vi "Window-Functional data editor.vi"(9 "Experiment Path":path=path "C:/Users/Teo/Desktop/UCL Datasets/160915_13_48_57 FunctAcq-6 patches", 11 "Standalone viewer?":bool=TRUE) -> ()   [LabVIEW 2020]
uses:
  User Interface/Visualisation/Timelapse Viewer/Typedefs/Custom slider-vertical.ctl
  User Interface/Visualisation/Timelapse Viewer/Typedefs/Colour.ctl
  User Interface/Visualisation/Timelapse Viewer/Typedefs/Channel to load.ctl
  User Interface/Visualisation/Timelapse Viewer/Typedefs/Time series viewer refs.ctl
  User Interface/Visualisation/Timelapse Viewer/Typedefs/Speed Viewer States enum.ctl
  <vilib>/Utility/miscctls.llb/LVPointTypeDef.ctl
  Typedefs/Save-Load enum.ctl
  <vilib>/vision/Image Controls.llb/IMAQ Image.ctl
  Typedefs/HW config states enum.ctl
  User Interface/Visualisation/Functional Imaging Viewer/Typedefs/Get-Set-Clear Control.ctl
  User Interface/Visualisation/Timelapse Viewer/Typedefs/Select Play-Stop button to show.ctl
  <vilib>/Utility/error.llb/DialogType.ctl
  User Interface/Visualisation/Timelapse Viewer/Cam video sync/Typedefs/Cam videos cluster.ctl
  User Interface/Visualisation/Timelapse Viewer/Globals/gl_Time series viewer globals.vi
  Global Variables/General Globals.vi
panel:
  in  "Channel to load":T1
  in  "Colour":T2
  in  "Number of rows to generate":i32=3 format="%.0f rows"
  in  "Source number of frames":T3(ring)=enum."As many as the number of cycles"
  out "Slider at frame #":i32 format="Cycle %.0f"
  in  "Scrollbar":i32(c297)
  in  "Back":bool
  in  "Play":bool
  in  "Stop":bool
  in  "Tab Control":enum32{"Camera videos", "Speed data"}(tab)
  out "Cams":T5 {"Vid4 Rel time (ms)" format="%.0f ms"; "Vid3 Rel time (ms)" format="%.0f ms"; "Vid2 Rel time (ms)" format="%.0f ms"; "Vid1 Rel time (ms)" format="%.0f ms"}
  out "Actual number \nof speed points":i32 format="Actual of speed points: %.0f"
  out "Speed Data":string[][](array[string])
  out "Expected speed values":dbl format="Expected speed points: %#_g"
  out "Original frame rate (fps)":dbl format="Original frame rate: %#.1f (fps)"
  out "Frame rate set (fps)":dbl format="Frame rate set: %#.1f (fps)"
  out "Actual frame rate (fps)":dbl format="Actual frame rate: %#.1f (fps)"
  out "AVI Mode ind":string="AVI mode:"
  out "Video length info":string="Duration: 00h 00m 00s, 0 frames"
  out "Export images":bool
  out "Export snippet":bool
  in  "Extraction Cursors":cluster{i32, i32}(slide)={1, 5594} scale=1.0..141.0
  out "Export vid":bool
  out "Stop (ind)":bool
  in  "Intensity":T6={0.0, 4095.0} scale=0.0..4095.0
  out "Speed Graph":dbl[](graph) caption="Speed Chart"
  out "Image":T4(plugin-control)
  # "Date                         Time                  Time stamp           Speed (rpm)          Angle (deg)"
  # "Timelapse Info"
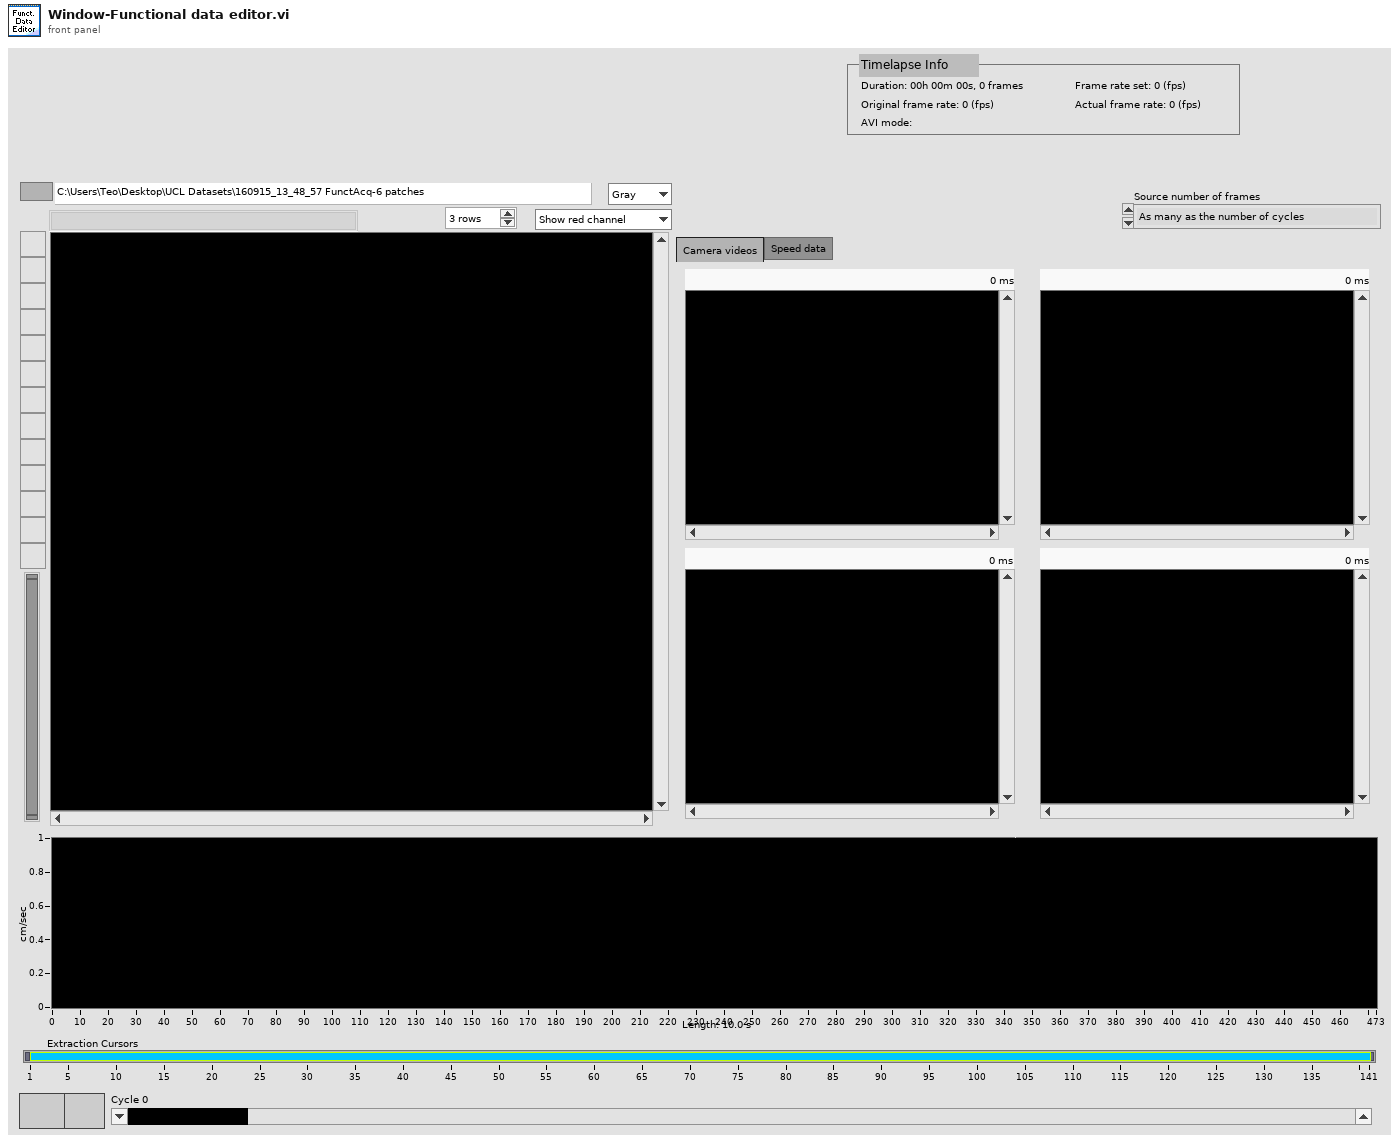
[diagram p1: front panel]
types:
  T1 = typedef "Channel to load.ctl" = enum16{"Show red channel", "Show green channel", "Show both channels"}
  T2 = typedef "Colour.ctl" = enum16{"Gray", "Red", "Green", "Mixed"}
  T3 = enum16{"As many as the frames in the video with the fewest frames", "As many as the number of cycles"}
  T4 = typedef "IMAQ Image.ctl" = refnum<image>
  T5 = cluster{"Vid 1":T4, "Vid 2":T4, "Vid 3":T4, "Vid 4":T4, "Vid1 Rel time (ms)":u32, "Vid2 Rel time (ms)":u32, "Vid3 Rel time (ms)":u32, "Vid4 Rel time (ms)":u32}
  T6 = typedef "Custom slider-vertical.ctl" = cluster{dbl, dbl}
  T7 = typedef "Time series viewer refs.ctl" = cluster{"This VI":refnum<vi>, "Image control":refnum<vi>, "AVI Mode ind":refnum<vi>, "Play":refnum<vi>, "Stop":refnum<vi>, "Back":refnum<vi>, "Scrollbar":refnum<vi>, "Video length info":refnum<vi>, "Expected speed values":refnum<vi>, "Intensity":refnum<vi>, "Path":refnum<vi>, "Selection sliders":refnum<vi>, "Speed Graph ref":refnum<vi>, "Frame rate set (fps)":refnum<vi>, "Number of rows to generate":refnum<vi>, "VL Image Array":refnum<vi>, "Image Scrollbar":refnum<vi>, "Channel to load":refnum<vi>, "Colour":refnum<vi>}
  T8 = typedef "Save-Load enum.ctl" = enum16{"Save to file", "Load from file", "Compare from file", "Save Backup"}
  T9 = enum16{"None", "Release queue", "Obtain queue", "Enqueue", "Get status", "Set status"}
  T10 = typedef "LVPointTypeDef.ctl" = cluster{"Horizontal":i16, "Vertical":i16}
  T11 = typedef "Speed Viewer States enum.ctl" = enum16{"Idle", "Initialise", "Playback", "Scroll bar event", "Speed cursor event", "Back to start", "Exit"}
  T12 = typedef "HW config states enum.ctl" = enum16{"Load from file", "Save to file", "Save backup", "Write all", "Read all", "Write XY stage settings", "Write DAQ FPGA settings", "Write Control FPGA settings", "Write Phys Channels", "Write System Config", "Write HW Config", "Save System Config", "Save HW Config", "Clear", "Compare from file"}
  T13 = typedef "Image Type" = u32
  T14 = typedef "Custom slider-horisontal.ctl" = cluster{dbl, dbl}
  T15 = typedef "Cam videos cluster.ctl" = cluster{"Vid 1":T4, "Vid 2":T4, "Vid 3":T4, "Vid 4":T4, "Vid1 Rel time (ms)":u32, "Vid2 Rel time (ms)":u32, "Vid3 Rel time (ms)":u32, "Vid4 Rel time (ms)":u32}
  T16 = typedef "Get-Set-Clear Control.ctl" = enum16{"Get", "Set", "Clear"}
  T17 = typedef "Select Play-Stop button to show.ctl" = enum16{"Show Play button", "Show Stop button"}
  T18 = typedef "DialogType.ctl" = u16
  T19 = typedef "Hardware Configuration settings.ctl" = cluster{"Dev. PC":bool, "Swap XY on stage":bool, "No of AOD":u8, "MC Supported":bool, "Axial MC":bool, "Computer MAC address":string, "Externalise Triggers":bool, "Trigger HW config":T20, "DAQmx Chan":T21, "XY stage available":bool, "XY Stage":T22, "Z stage available":bool, "Z Stage config cluster":T23, "Encoder available":bool, "Encoder":T24, "VidRec available":bool, "Cam VidRec":T25, "Laser Power Control HW config":T26, "Laser 1 available":bool, "Laser 1 config cluster":T27, "Prechirper 1 available":bool, "Prechirper 1 config cluster":T28, "Control system.FPGA available?":bool, "Control Sys. HW config":T29, "DAQ FPGA HW Config":T30, "PMT Voltage Range":T34}
  T20 = typedef "Triggers HW config.ctl" = cluster{"Available Device List":i32, "Device Address":string}
  T21 = typedef "DAQmx physical channels cluster.ctl" = cluster{"Pockels AO":tag, "Hard shutter AO":tag, "PMT AOs":tag, "Galvo AOs":tag, "Power meter AI":tag}
  T22 = typedef "XY Stage config cluster.ctl" = cluster{"COM port":refnum<visa-resource-name>, "Baudrate":i32, "Type":string}
  T23 = typedef "Z Stage config cluster.ctl" = cluster{"COM port":refnum<visa-resource-name>, "Baudrate":i32, "Type":string}
  T24 = typedef "Encoder config cluster.ctl" = cluster{"IP address":string, "Port":u16, "Wheel radius (cm)":dbl, "Encoder Trigger":tag}
  T25 = typedef "Cam VidRec HW config setup cluster.ctl" = cluster{"DO flag-Video record":tag, "DO flag-Trial start":tag}
  T26 = typedef "Laser Power Control HW config.ctl" = cluster{"Laser Power Control":string, "Laser Power Modulation Control":enum16{"NI", "FPGA"}}
  T27 = typedef "Laser 1 config cluster.ctl" = cluster{"COM port":refnum<visa-resource-name>, "Baud Rate":i32, "Type":string}
  T28 = typedef "PreChirper 1 config cluster.ctl" = cluster{"Type":string, "Baud Rate":i32, "COM port":refnum<visa-resource-name>}
  T29 = typedef "Control Sys HW config cluster.ctl" = cluster{"Control system.FPGA Type":enum16{"Virtex 5", "Virtex 7"}, "Control system.Network adapter name":string, "Control system.MAC address":string, "Control system.Ethernet Port":u32, "Control system.Ethernet Port Opened":bool}
  T30 = typedef "DAQ FPGA HW config cluster.ctl" = cluster{"FGPA Ref":T31, "Target":T32, "input card type":T33}
  T31 = typedef "FPGA Ref.ctl" = refnum<k20>
  T32 = typedef "nirio_resource_hc.ctl" = tag
  T33 = typedef "FPGA input type AC-DC.ctl" = enum16{"AC Card", "DC Card"}
  T34 = typedef "PMT Voltage Range.ctl" = cluster{"PMT Voltage Lower Limit":dbl, "PMT Voltage Upper Limit":dbl}
  T35 = cluster{"Start Frame No":i32, "End Frame No":i32}
  T36 = typedef "IMAQ AVI2 Refnum.ctl" = refnum<k20>
  T37 = cluster{"# of frames to export":i32, "Initial frame's owning file":T36, "8-bit AVI file path":path, "Cursors location":cluster{"Number of first frame":i32, "Number of last frame":i32}}
  T38 = enum32{"Invalid", "Standard", "Closed", "Hidden", "Minimized", "Maximized"}
  T39 = typedef "Speed graph behaviour enum.ctl" = enum16{"Scrolling data", "Scrolling cursor"}
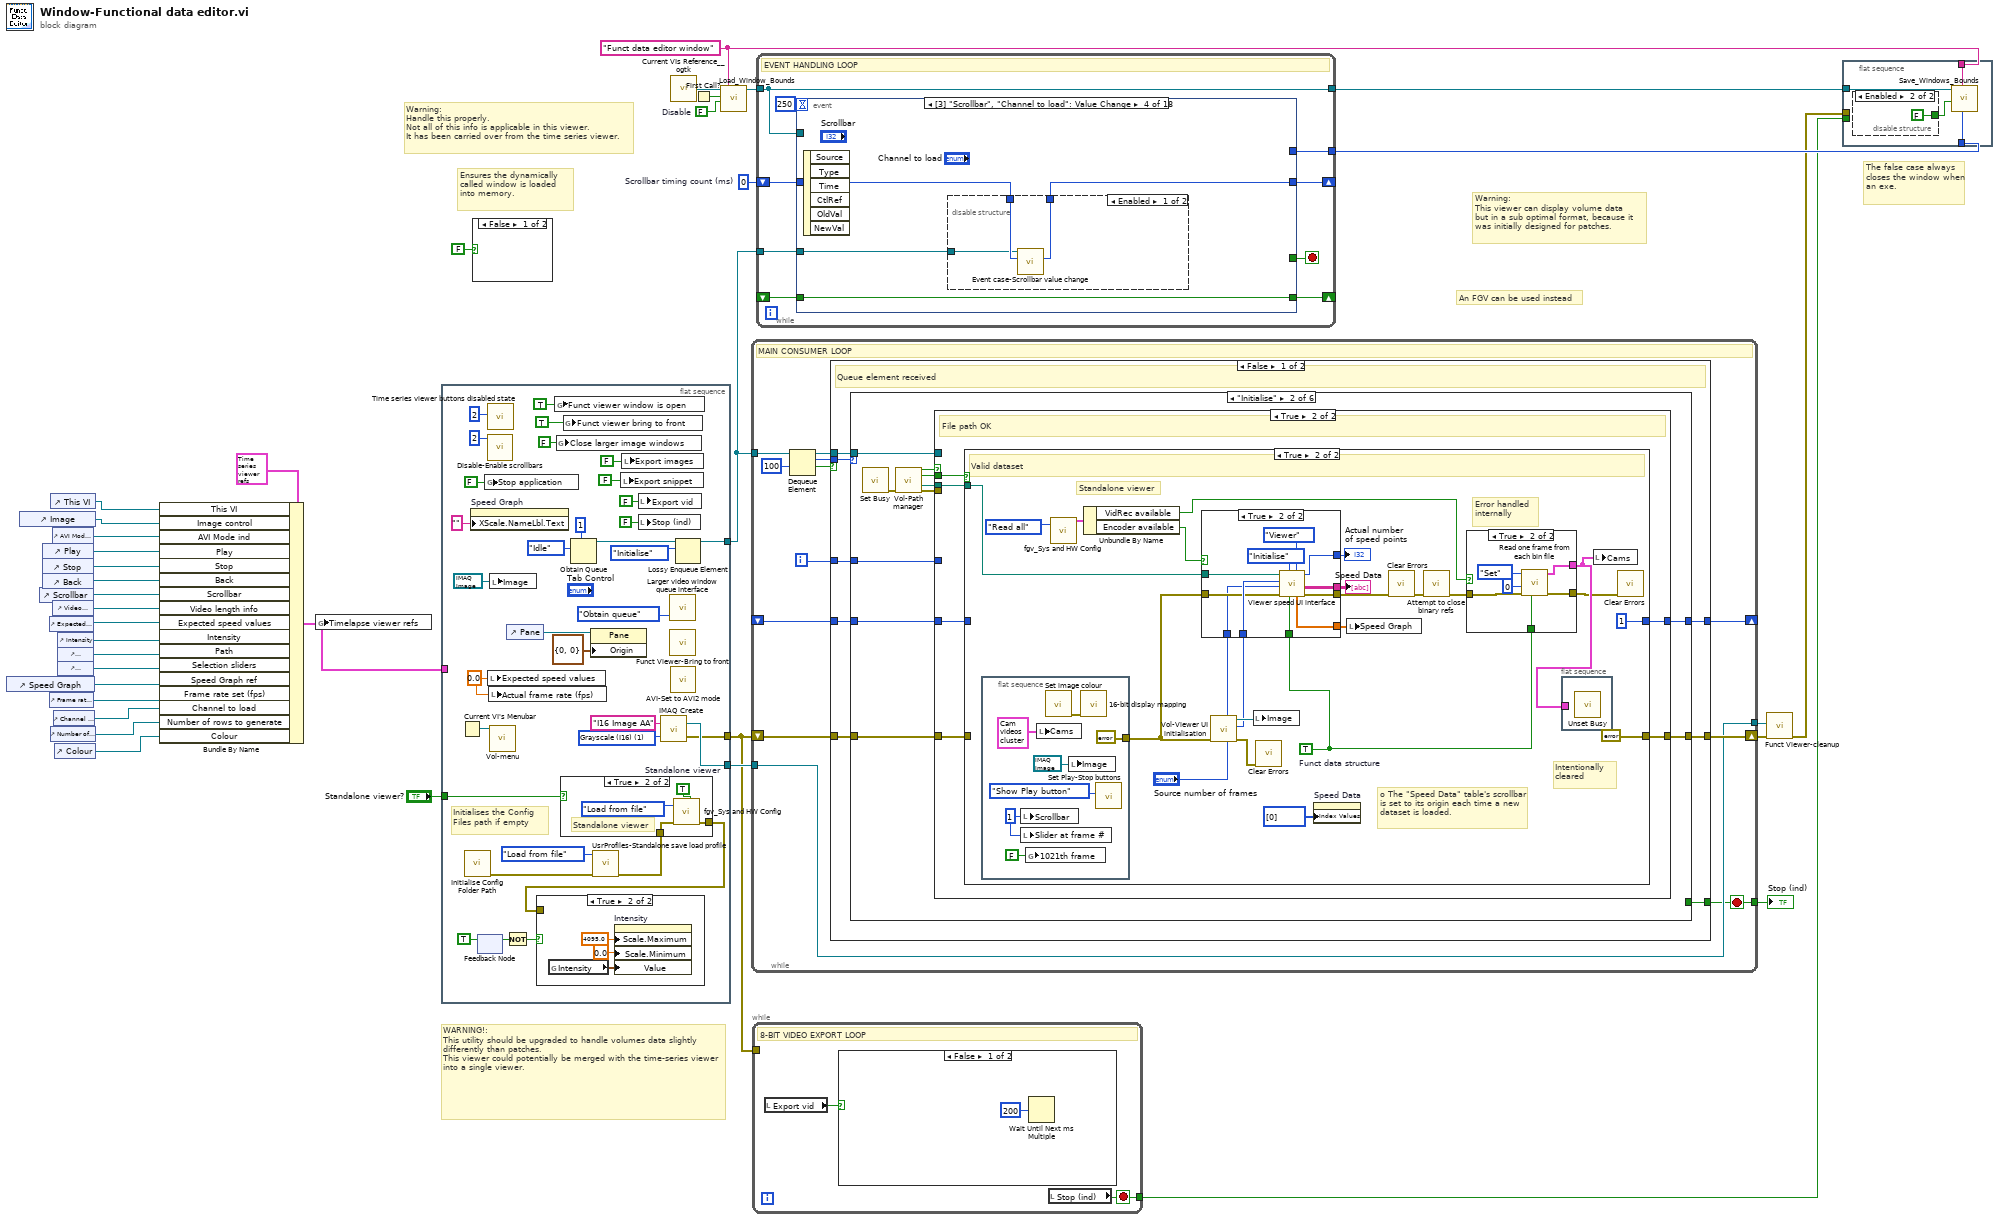
[diagram p0: block diagram]
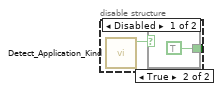
[diagram p2: hidden frame]
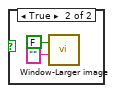
[diagram p4: hidden frame]
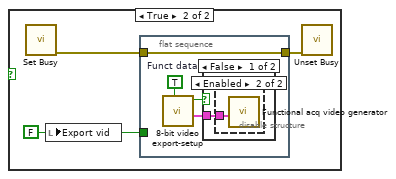
[diagram p5: hidden frame]
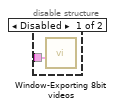
[diagram p6: hidden frame]
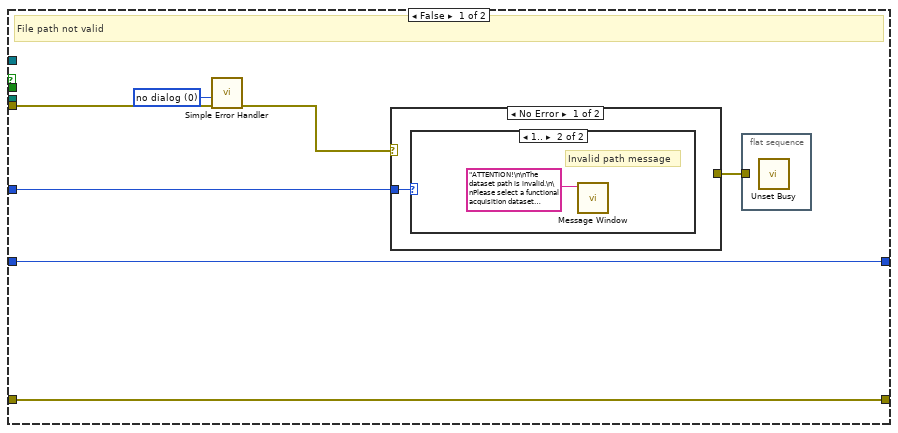
[diagram p11: hidden frame]
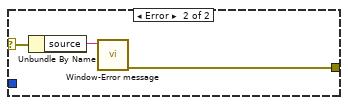
[diagram p13: hidden frame]
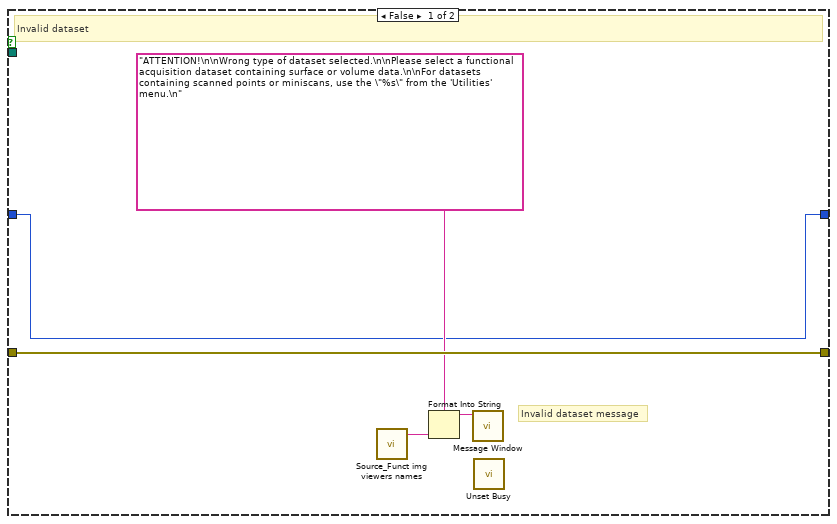
[diagram p14: hidden frame]
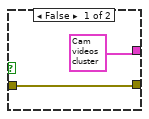
[diagram p15: hidden frame]
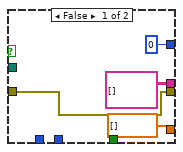
[diagram p16: hidden frame]
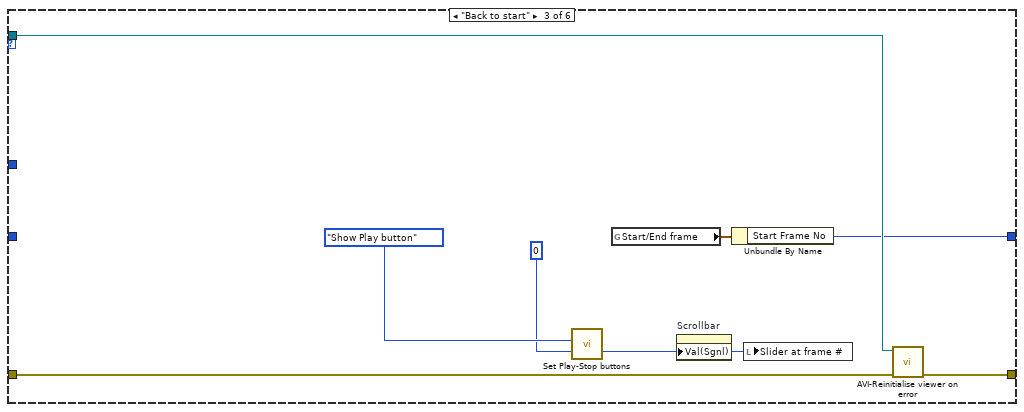
[diagram p17: hidden frame]
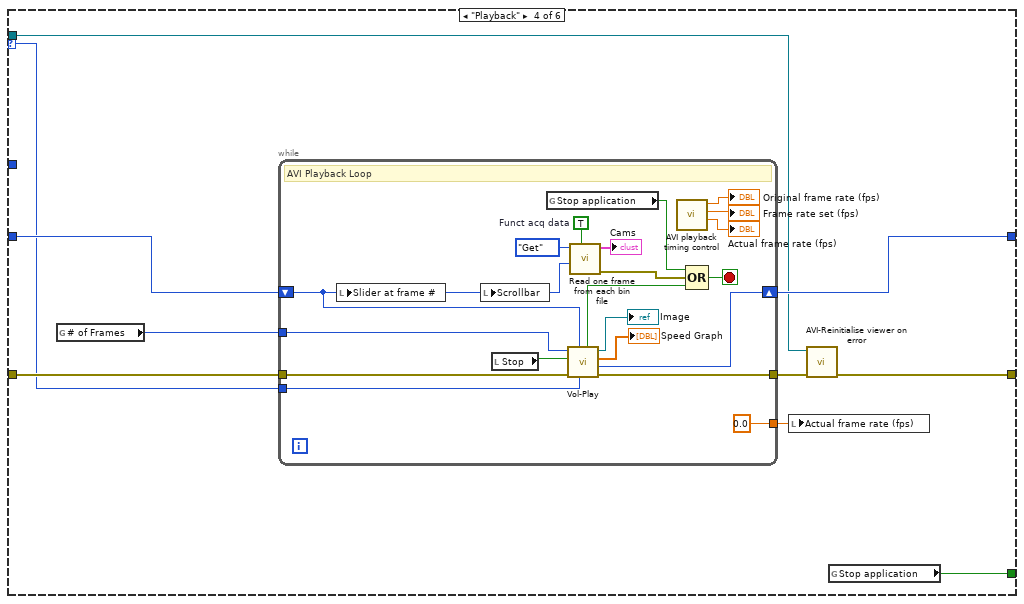
[diagram p18: hidden frame]
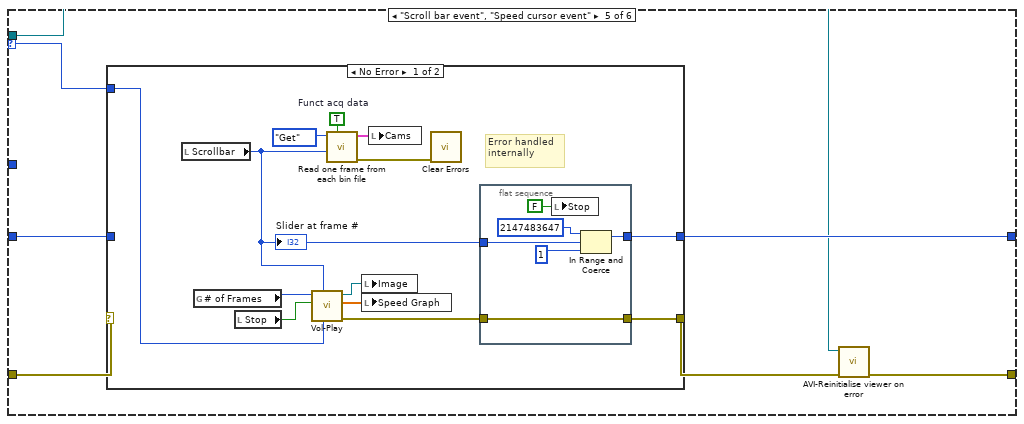
[diagram p19: hidden frame]
diagram:
  w15 = FALSE  # Disable
  w14 = "Funct data editor window" ("Window Name (i.e. Key)")
  w24 = u32 0  # Scrollbar timing count (ms)
  # "Warning:\nThis viewer can display volume data\nbut in a sub optimal format, because it\nwas initially designed for patches."
  # "Warning:\nHandle this properly.\nNot all of this info is applicable in this viewer.\nIt has been carried over from the time series viewer."
  # "WARNING!:\nThis utility should be upgraded to handle volumes data slightly differently than patches.\nThis viewer could potentially be merged with the time-series viewer into a single viewer."
  # "The false case always closes the window when an exe."
  # "Ensures the dynamically called window is loaded into memory."
  # "An FGV can be used instead"
  n1 = control-ref of="Speed Graph"() -> (w19:refnum<vi>)
  n2 = control-ref of="Image"() -> (w4:refnum<vi>)
  n3 = control-ref of="Scrollbar"() -> (w28:refnum<vi>)
  n4 = control-ref of="Play"() -> (w31:refnum<vi>)
  n5 = control-ref of="Stop"() -> (w30:refnum<vi>)
  n6 = control-ref of="Back"() -> (w29:refnum<vi>)
  n7 = control-ref of="Expected speed values"() -> (w26:refnum<vi>)
  n8 = control-ref of="Frame rate set (fps)"() -> (w8:refnum<vi>)
  n9 = control-ref of="This VI"() -> (w22:refnum<vi>)
  n10 = control-ref of="Number of rows to generate"() -> (w6:refnum<vi>)
  n11 = control-ref of="AVI Mode ind"() -> (w34:refnum<vi>)
  n12 = control-ref of="Video length info"() -> (w27:refnum<vi>)
  n13 = control-ref of="Channel to load"() -> (w2:refnum<vi>)
  n14 = control-ref of="Colour"() -> (w1:refnum<vi>)
  n15 = control-ref of="Intensity"() -> (w25:refnum<vi>)
  n16 = control-ref of="Experiment Path"() -> (w23:refnum<vi>)
  n17 = control-ref of="Extraction Cursors"() -> (w20:refnum<vi>)
  n18 = Bundle By Name(cluster=T7 {"This VI"=refnum, "Image control"=refnum, "AVI Mode ind"=refnum, "Play"=refnum, "Stop"=refnum, "Back"=refnum, "Scrollbar"=refnum, "Video length info"=refnum, "Expected speed values"=refnum, "Intensity"=refnum, "Path"=refnum, "Selection sliders"=refnum, "Speed Graph ref"=refnum, "Frame rate set (fps)"=refnum, "Number of rows to generate"=refnum, "VL Image Array"=refnum, "Image Scrollbar"=refnum, "Channel to load"=refnum, "Colour"=refnum}, "This VI"=w22, "Image control"=w4, "AVI Mode ind"=w34, "Play"=w31, "Stop"=w30, "Back"=w29, "Scrollbar"=w28, "Video length info"=w27, "Expected speed values"=w26, "Intensity"=w25, "Path"=w23, "Selection sliders"=w20, "Speed Graph ref"=w19, "Frame rate set (fps)"=w8, "Channel to load"=w2, "Number of rows to generate"=w6, "Colour"=w1) -> (w3:T7)
  n19 = global write "gl_Time series viewer globals.vi" "Timelapse viewer refs"(w3) -> ()
  n20 = flat-sequence {
    tunnel: [w69] -> w37
    tunnel: [w42] -> w18
    tunnel: [w66] -> w35
    tunnel: w3 -> [_]
    tunnel: "Standalone viewer?" -> [w41]
    frame #0 {
      w62 = 0.0 ("Expected speed points")
      w71 = T13 1 items=["Grayscale (U8)", "Grayscale (I16)", "Grayscale (SGL)", "Complex (CSG)", "RGB (U32)", "HSL (U32)", "RGB (U64)", "Grayscale (U16)"] ("Image Type")
      # "Initialises the Config Files path if empty"
      n21 = Current VI's Menubar() -> (w61:refnum<k9>)
      n22 = call "Initialise Config Folder Path.vi"() -> ("error out"=w47:errorcluster)  [unwired: 9 in, 2 out]
      n23 = property on="Speed Graph" class="WFGraph (strict)"("XScale.NameLbl.Text"="" ("X Scale.Name Label.Text")) -> ()  [unwired: 2 in, 2 out]
      n24 = feedback #1() -> (w43:bool)  [unwired: 1 in]
      n25 = feedback-in #1(TRUE) -> ()
      n26 = global write "General Globals.vi" "Stop application"(FALSE ("Stop application")) -> ()
      n27 = call "Disable-Enable scrollbars.vi"("Disabled state"=2) -> ()  [unwired: 10 in, 1 out]
      n28 = call "Time series viewer buttons disabled state.vi"("Disabled"=2) -> ()  [unwired: 10 in, 1 out]
      n29 = local write "Expected speed values"(w62) -> ()
      n30 = local write "Actual frame rate (fps)"(w62) -> ()
      n31 = local write "Image"(T4 refnum ("Image")) -> ()
      n32 = call "Vol-menu.vi"("menu"=w61) -> ()  [unwired: 9 in, 2 out]
      n33 = Not(x=w43) -> (.not. x?=w45:bool)
      n34 = control-ref of="Pane"() -> (w63:refnum<vi>)
      n35 = global write "gl_Time series viewer globals.vi" "Funct viewer window is open"(TRUE ("Bring Timelapse Editor to front")) -> ()
      n36 = global write "gl_Time series viewer globals.vi" "Close larger image windows"(FALSE ("Close larger image window")) -> ()
      n37 = global write "gl_Time series viewer globals.vi" "Funct viewer bring to front"(TRUE ("Window is open")) -> ()
      n38 = Obtain Queue(max queue size (-1, unlimited)=1, element data type=Speed_Viewer_States_enum."Idle" ("States")) -> (queue out=w67:refnum<queue>)  [unwired: 3 in, 2 out]
      n39 = property class="Pane"(reference=w63, "Origin"=T10 {"Horizontal"=0, "Vertical"=0}) -> ()  [unwired: 1 in, 2 out]
      n40 = call "UsrProfiles-Standalone save load profile.vi"("Error in"=w47, "Function"=Save-Load_enum."Load from file") -> ("error out"=w40:errorcluster)  [unwired: 9 in]
      n41 = case shown="True" w41 {
        tunnel: w40 -> [w72 w75]
        tunnel: [w72 w74] -> w39
        frame False {
          # "No need to load the system\nconfig. Already loaded."
        }
        frame True {
          w73 = TRUE  # Standalone viewer
          # "Standalone viewer"
          n42 = call "fgv_Sys and HW Config.vi"("Standalone viewer initialisation?"=w73, "Function"=HW_config_states_enum."Load from file", "error in (no error)"=w75) -> ("error out"=w74:errorcluster)  [unwired: 6 in, 2 out]
        }
      }
      n43 = case shown="True" w45 {
        tunnel: w39 -> [_ _]
        frame False {
        }
        frame True {
          n44 = global read "gl_Time series viewer globals.vi" "Intensity"() -> (w77:T14)
          n45 = property on="Intensity" class="Slide (strict)"("Scale.Maximum"=4095.0 ("Scale.Range:Maximum"), "Scale.Minimum"=0.0 ("Scale.Range:Minimum"), "Value"=w77) -> ()  [unwired: 2 in, 2 out]
        }
      }
      n46 = local write "Export snippet"(FALSE ("Export data subset")) -> ()
      n47 = local write "Export images"(FALSE ("Export data subset")) -> ()
      n48 = local write "Export vid"(FALSE ("Export")) -> ()
      n49 = local write "Stop (ind)"(FALSE ("Boolean")) -> ()
      n50 = call "IMAQ Create"("Image Name"="I16 Image AA", "Image Type"=w71) -> ("New Image"=w69:T4, "error out"=w42:errorcluster)  [unwired: 2 in, 1 out]
      n51 = call "Larger video window queue interface.vi"("Function"=T9."Obtain queue") -> ()  [unwired: 10 in, 1 out]
      n52 = call "Funct Viewer-Bring to front.vi"() -> ()  [unwired: 12 in]
      n53 = call "AVI-Set to AVI2 mode.vi"() -> ()  [unwired: 11 in, 1 out]
      n54 = Lossy Enqueue Element(queue=w67, element=Speed_Viewer_States_enum."Initialise" ("States")) -> (queue out=w66:refnum<queue>)  [unwired: 1 in, 3 out]
    }
  }
  n55 = case shown="False" FALSE {
    frame False {
    }
    frame True {
      n56 = call "Window-Larger image.vi"("Image name"="", "Open maximised"=FALSE) -> ()  [unwired: 10 in]
    }
  }
  n57 = call <userlib>:"Current VIs Reference__ogtk.vi"() -> ("Current VI's reference"=w17:refnum<vi>)  [unwired: 5 in]
  n58 = First Call?() -> (First Call?: T/F=w16:bool)
  n59 = call "Load_Window_Bounds.vi"("Window Name (i.e. Key)"=w14, "Disable"=w15, "First Call"=w16, "Window VI's Ref"=w17) -> ("reference out"=w11:refnum<vi>)  [unwired: 4 in, 3 out]
  n60 = while {
    tunnel: w37 -> [w85]
    tunnel: [w85] -> w36
    shift-right: [w91] -> _
    shift-left: _ -> [w90]
    tunnel: w35 -> [w89]
    shift-right: [w92] -> w32
    shift-left: w18 -> [w93]
    tunnel: [w84] -> w21
    i -> [w83]
    stop <- w84 stop-if-true
    # "MAIN CONSUMER LOOP"
    n61 = Dequeue Element(queue=w89, timeout in ms (-1)=100) -> (queue out=w82:refnum<queue>, element=w86:T11, timed out?=w87:bool)  [unwired: 1 in, 1 out]
    n62 = case shown="False" w87 {
      tunnel: w93 -> [w101 w262]
      tunnel: [w100 w262] -> w92
      tunnel: [w99 w263] -> w91
      tunnel: w90 -> [w98 w263]
      tunnel: w86 -> [w97 _]
      tunnel: [w96 w261] -> w84
      tunnel: w82 -> [w95 _]
      tunnel: w83 -> [w94 _]
      frame False {
        # "Queue element received"
        n63 = case shown="\"Initialise\"" w97 {
          selector: w97 -> [_ _ _ w198 w228 _]
          tunnel: w101 -> [w102 w113 w196 w207 w233 w256]
          tunnel: [w102 w112 w195 w204 w231 w256] -> w100
          tunnel: [w103 w114 w192 w206 w234 1 ("Slide")] -> w99
          tunnel: w98 -> [w103 w111 _ w205 w232 _]
          tunnel: [_ _ _ w199 _ TRUE] -> w96
          tunnel: w95 -> [_ w110 w194 w202 w229 _]
          tunnel: w94 -> [_ w109 _ _ _ _]
          frame Default {
          }
          frame "Initialise" {
            n64 = call <vilib>:"Set Busy.vi"() -> ("error out"=w105:errorcluster)  [unwired: 10 in, 1 out]
            n65 = call "Vol-Path manager.vi"("error in (no error)"=w105) -> ("File path OK"=w108:bool, "Valid data type (& valid path)"=w104:bool, "Speed Data folder path+dummy filename"=w107:path, "error"=w106:errorcluster)  [unwired: 10 in, 1 out]
            n66 = case shown="True" w108 {
              tunnel: [w121 w130] -> w114
              tunnel: w107 -> [_ w131]
              tunnel: w113 -> [w120 w127]
              tunnel: [w120 w132] -> w112
              tunnel: w111 -> [w121 w128]
              tunnel: w106 -> [w119 _]
              tunnel: w110 -> [_ _]
              tunnel: w109 -> [w116 _]
              tunnel: w104 -> [_ w129]
              frame False {
                w118 = T18 0 items=["no dialog", "OK message", "continue or stop message", "OK message + warnings", "continue/stop + warnings"] ("type of dialog (OK msg:1)")
                # "File path not valid"
                n67 = call <vilib>:"Simple Error Handler.vi"("type of dialog (OK msg:1)"=w118, "error in (no error)"=w119) -> ("error out"=w117:errorcluster)  [unwired: 3 in, 4 out]
                n68 = case shown="No Error" w117 {
                  selector: w117 -> [_ w126]
                  tunnel: w116 -> [w122 _]
                  tunnel: [_ w124] -> w115
                  frame No Error {
                    n69 = case shown="1.." w122 {
                      frame 0, Default {
                      }
                      frame 1.. {
                        # "Invalid path message"
                        n70 = call "Message Window.vi"("Message string"="ATTENTION!\n\nThe dataset path is invalid.\n\nPlease select a functional acquisition dataset containing surface or volume data.\n") -> ()  [unwired: 10 in, 1 out]
                      }
                    }
                  }
                  frame Error {
                    n71 = Unbundle By Name(w126) -> ("source"=w125:string)
                    n72 = call "Window-Error message.vi"("Message"=w125) -> ("Error Out (no error)"=w124:errorcluster)  [unwired: 10 in]
                  }
                }
                n73 = flat-sequence {
                  tunnel: w115 -> [_]
                  frame #0 {
                    n74 = call <vilib>:"Unset Busy.vi"() -> ()  [unwired: 11 in, 1 out]
                  }
                }
              }
              frame True {
                # "File path OK"
                n75 = case shown="True" w129 {
                  tunnel: [w137 errorcluster {"status"=FALSE, "code"=0, "source"=""} ("error out")] -> w132
                  tunnel: w131 -> [_ w159]
                  tunnel: [w134 1 ("Slide")] -> w130
                  tunnel: w128 -> [w134 _]
                  tunnel: w127 -> [w137 _]
                  frame False {
                    # "Invalid dataset message"
                    # "Invalid dataset"
                    n76 = call "Source_Funct img viewers names.vi"() -> ("Name string: Functional imaging viewer (POI/Mscn)"=w135:string)  [unwired: 10 in, 1 out]
                    n77 = Format Into String(format string="ATTENTION!\n\nWrong type of dataset selected.\n\nPlease select a functional acquisition dataset containing surface or volume data.\n\nFor datasets containing scanned points or miniscans, use the \"%s\" from the 'Utilities' menu.\n" ("Message"), w135) -> (resulting string=w133:string)  [unwired: 2 in, 1 out]
                    n78 = call "Message Window.vi"("Message string"=w133) -> ()  [unwired: 10 in, 1 out]
                    n79 = call <vilib>:"Unset Busy.vi"() -> ()  [unwired: 11 in, 1 out]
                  }
                  frame True {
                    w143 = TRUE  # Funct data structure
                    # "Standalone viewer"
                    # "o\tThe \"Speed Data\" table's scrollbar is set to its origin each time a new dataset is loaded."
                    # "Error handled internally"
                    # "Intentionally cleared"
                    # "Valid dataset"
                    n80 = flat-sequence {
                      tunnel: [errorcluster {"status"=FALSE, "code"=0, "source"=""} ("error out")] -> w150
                      frame #0 {
                        w185 = 1 ("Scrollbar")
                        n81 = local write "Scrollbar"(w185) -> ()
                        n82 = local write "Slider at frame #"(w185) -> ()
                        n83 = global write "gl_Time series viewer globals.vi" "1021th frame"(FALSE ("1021th frame")) -> ()
                        n84 = local write "Cams"(T15 {"Vid 1"=refnum, "Vid 2"=refnum, "Vid 3"=refnum, "Vid 4"=refnum, "Vid1 Rel time (ms)"=0, "Vid2 Rel time (ms)"=0, "Vid3 Rel time (ms)"=0, "Vid4 Rel time (ms)"=0} ("Cam videos cluster")) -> ()
                        n85 = call "Set image colour.vi"() -> ("error out"=w184:errorcluster)  [unwired: 11 in]
                        n86 = local write "Image"(T4 refnum ("New Image")) -> ()
                        n87 = call "16-bit display mapping.vi"("error in (no error)"=w184) -> ()  [unwired: 10 in, 1 out]
                        n88 = call "Set Play-Stop buttons.vi"("Function"=Select_Play-Stop_button_to_show."Show Play button") -> ()  [unwired: 10 in, 1 out]
                      }
                    }
                    n89 = call "fgv_Sys and HW Config.vi"("Function"=HW_config_states_enum."Read all") -> ("Hardware Configuration OUT"=w140:T19)  [unwired: 8 in, 2 out]
                    n90 = Unbundle By Name(w140) -> ("VidRec available"=w138:bool, "Encoder available"=w139:bool)
                    n91 = call "Vol-Viewer UI initialisation.vi"("Source number of frames"="Source number of frames", "error in (no error)"=w150) -> ("error out"=w145:errorcluster, "Number of Frames"=w155:u32, "Image ref"=w156:T4, "Scrollbar position"=w144:i32)  [unwired: 5 in, 1 out]
                    n92 = case shown="True" w139 {
                      tunnel: w159 -> [_ w183]
                      tunnel: [dbl[] [] ("Speed waveform graph data") w182] -> w157
                      tunnel: w155 -> [_ w181]
                      tunnel: [string[][] [] ("Speed Data") w180] -> w154
                      tunnel: [w170 w179] -> w153
                      tunnel: w150 -> [w170 w178]
                      tunnel: [0 ("Actual number of speed values") w176] -> w148
                      tunnel: w144 -> [_ w175]
                      tunnel: w143 -> [_ w173]
                      frame False {
                      }
                      frame True {
                        n93 = call "Viewer speed UI interface.vi"("Caller"=enum16{"Viewer", "Exporter"}."Viewer", "Funct data structure"=w173, "Function"=enum16{"Initialise", "Update"}."Initialise", "error in (no error)"=w178, "Gobal frame number in Timelapse data/master video (1 based)"=w175, "Number of Frames"=w181, "Speed Data folder path+dummy filename"=w183) -> ("error out"=w179:errorcluster, "Speed Data"=w180:string[][], "Actual number of speed values"=w176:i32, "Speed waveform graph data"=w182:dbl[])  [unwired: 1 in]
                      }
                    }
                    "Speed Data" <- w154
                    "Actual number \nof speed points" <- w148
                    n94 = local write "Image"(w156) -> ()
                    n95 = call <vilib>:"Clear Errors.vi"("error in (no error)"=w145) -> ()  [unwired: 5 in, 2 out]
                    n96 = property on="Speed Data" class="Arr (strict)"("Index Values"=u32[] [0]) -> ()  [unwired: 2 in, 2 out]
                    n97 = local write "Speed Graph"(w157) -> ()
                    n98 = call <vilib>:"Clear Errors.vi"("error in (no error)"=w153) -> ("error out"=w151:errorcluster)  [unwired: 5 in, 1 out]
                    n99 = call "Attempt to close binary refs.vi"("error in (no error)"=w151) -> ("error out"=w152:errorcluster)  [unwired: 10 in]
                    n100 = case shown="True" w138 {
                      tunnel: w152 -> [w162 w166]
                      tunnel: [T15 {"Vid 1"=refnum, "Vid 2"=refnum, "Vid 3"=refnum, "Vid 4"=refnum, "Vid1 Rel time (ms)"=0, "Vid2 Rel time (ms)"=0, "Vid3 Rel time (ms)"=0, "Vid4 Rel time (ms)"=0} ("Cam videos cluster") w165] -> w149
                      tunnel: [w162 w164] -> w146
                      tunnel: w143 -> [_ w163]
                      frame False {
                      }
                      frame True {
                        n101 = call "Read one frame from each bin file.vi"("Funct data structure"=w163, "error in (no error)"=w166, "Master video's frame number (unity-based)"=0 ("Frame number"), "Get/set"=Get-Set-Clear_Control."Set" ("GEt set .bin refs")) -> ("Error out"=w164:errorcluster, "Cam videos cluster"=w165:T15)  [unwired: 6 in]
                      }
                    }
                    n102 = flat-sequence {
                      tunnel: w149 -> [_]
                      frame #0 {
                        n103 = call <vilib>:"Unset Busy.vi"() -> ()  [unwired: 11 in, 1 out]
                      }
                    }
                    n104 = local write "Cams"(w149) -> ()
                    n105 = call <vilib>:"Clear Errors.vi"("error in (no error)"=w146) -> ()  [unwired: 5 in, 2 out]
                  }
                }
              }
            }
          }
          frame "Back to start" {
            w191 = 0 ("Scrollbar")
            n106 = call "Set Play-Stop buttons.vi"("Function"=Select_Play-Stop_button_to_show."Show Play button") -> ()  [unwired: 10 in, 1 out]
            n107 = global read "gl_Time series viewer globals.vi" "Start/End frame"() -> (w193:T35)
            n108 = property on="Scrollbar" class="Scroll (strict)"("Val(Sgnl)"=w191) -> ()  [unwired: 2 in, 2 out]
            n109 = Unbundle By Name(w193) -> ("Start Frame No"=w192:i32)
            n110 = local write "Slider at frame #"(w191) -> ()
            n111 = call "AVI-Reinitialise viewer on error.vi"("error in (no error)"=w196, "Queue in"=w194) -> ("error out"=w195:errorcluster)  [unwired: 9 in]
          }
          frame "Playback" {
            n112 = global read "gl_Time series viewer globals.vi" "# of Frames"() -> (w201:u32)
            n113 = while {
              tunnel: w207 -> [w226]
              tunnel: [w227] -> w203
              shift-right: [w224] -> w206
              shift-left: w205 -> [w215]
              tunnel: w201 -> [w219]
              tunnel: [0.0 ("Expected speed points")] -> w200
              tunnel: w198 -> [w208]
              stop <- w212 stop-if-true
              w209 = TRUE  # Funct acq data
              # "AVI Playback Loop"
              n114 = local write "Slider at frame #"(w215) -> ()
              n115 = local write "Scrollbar"(w215) -> ()
              n116 = local read "Stop"() -> (w220:bool)
              n117 = global read "General Globals.vi" "Stop application"() -> (w210:bool)
              n118 = call "Vol-Play.vi"("State"=w208, "Cycle number (in)"=w215, "error in (no error)"=w226, "Stop button pressed"=w220, "Number of Frames"=w219) -> ("error out"=w227:errorcluster, "Cycle number (out)"=w224:i32, "Speed data waveform graph"=→"Speed Graph":dbl[], "I mage ref out"=→"Image":T4, "Playback stopped"=w213:bool)  [unwired: 1 in, 1 out]
              n119 = call "Read one frame from each bin file.vi"("Funct data structure"=w209, "Master video's frame number (unity-based)"=w215, "Get/set"=Get-Set-Clear_Control."Get" ("GEt set .bin refs")) -> ("Error out"=w211:errorcluster, "Cam videos cluster"=→"Cams":T15)  [unwired: 7 in]
              n120 = call "AVI playback timing control.vi"() -> ("Actual frame rate (fps)"=→"Actual frame rate (fps)":dbl, "Frame rate set OR original (fps)"=→"Frame rate set (fps)":dbl, "Original frame rate (fps)"=→"Original frame rate (fps)":dbl)  [unwired: 8 in, 1 out]
              n121 = Compound Arithmetic op=OR(w210, w211, w213) -> (w212:bool)
            }
            n122 = local write "Actual frame rate (fps)"(w200) -> ()
            n123 = call "AVI-Reinitialise viewer on error.vi"("error in (no error)"=w203, "Queue in"=w202) -> ("error out"=w204:errorcluster)  [unwired: 9 in]
            n124 = global read "General Globals.vi" "Stop application"() -> (w199:bool)
          }
          frame "Scroll bar event", "Speed cursor event" {
            n125 = case shown="No Error" w233 {
              selector: w233 -> [_ w255]
              tunnel: [w247 w254] -> w234
              tunnel: [w244 w255] -> w230
              tunnel: w232 -> [_ w254]
              tunnel: w228 -> [w243 _]
              frame No Error {
                w239 = TRUE  # Funct acq data
                # "Error handled internally"
                n126 = local read "Scrollbar"() -> (w246:i32)
                "Slider at frame #" <- w246
                n127 = global read "gl_Time series viewer globals.vi" "# of Frames"() -> (w237:u32)
                n128 = local read "Stop"() -> (w236:bool)
                n129 = call "Vol-Play.vi"("State"=w243, "Cycle number (in)"=w246, "Stop button pressed"=w236, "Number of Frames"=w237) -> ("error out"=w245:errorcluster, "Speed data waveform graph"=w238:dbl[], "I mage ref out"=w235:T4)  [unwired: 2 in, 3 out]
                n130 = call "Read one frame from each bin file.vi"("Funct data structure"=w239, "Master video's frame number (unity-based)"=w246, "Get/set"=Get-Set-Clear_Control."Get" ("GEt set .bin refs")) -> ("Error out"=w240:errorcluster, "Cam videos cluster"=w242:T15)  [unwired: 7 in]
                n131 = local write "Image"(w235) -> ()
                n132 = local write "Speed Graph"(w238) -> ()
                n133 = local write "Cams"(w242) -> ()
                n134 = call <vilib>:"Clear Errors.vi"("error in (no error)"=w240) -> ()  [unwired: 5 in, 2 out]
                n135 = flat-sequence {
                  tunnel: [w251] -> w247
                  tunnel: w246 -> [w249]
                  tunnel: [w248] -> w244
                  tunnel: w245 -> [w248]
                  frame #0 {
                    n136 = local write "Stop"(FALSE ("Stop")) -> ()
                    n137 = In Range and Coerce(upper limit=2147483647, x=w249, lower limit=1) -> (coerced(x)=w251:i32)  [unwired: 1 out]
                  }
                }
              }
              frame Error {
              }
            }
            n138 = call "AVI-Reinitialise viewer on error.vi"("error in (no error)"=w230, "Queue in"=w229) -> ("error out"=w231:errorcluster)  [unwired: 9 in]
          }
          frame "Exit" {
            n139 = local read "Stop"() -> (w259:bool)
            n140 = case shown="True" w259 {
              frame False {
              }
              frame True {
                n141 = local write "Stop"(FALSE ("Stop")) -> ()
              }
            }
          }
        }
      }
      frame True {
        # "Timeout"
        n142 = global read "General Globals.vi" "Stop application"() -> (w261:bool)
      }
    }
  }
  "Stop (ind)" <- w21
  n143 = while {
    tunnel: w18 -> [_]
    tunnel: [w264] -> w7
    stop <- w264 stop-if-true
    # "8-BIT VIDEO EXPORT LOOP"
    n144 = local read "Export vid"() -> (w265:bool)
    n145 = case shown="False" w265 {
      frame False {
        n146 = Wait Until Next ms Multiple(millisecond multiple=u32 200) -> ()  [unwired: 1 out]
      }
      frame True {
        w269 = FALSE ("Export")
        n147 = call <vilib>:"Set Busy.vi"() -> ("error out"=w268:errorcluster)  [unwired: 10 in, 1 out]
        n148 = local write "Export vid"(w269) -> ()
        n149 = flat-sequence {
          tunnel: w269 -> [_]
          tunnel: w268 -> [w273]
          tunnel: [w273] -> w267
          frame #0 {
            w270 = TRUE  # Funct data
            n150 = call "8-bit video export-setup.vi"("Funct data?"=w270) -> ("output cluster"=w272:T37, "cancelled"=w271:bool)  [unwired: 8 in, 1 out]
            n151 = case shown="False" w271 {
              tunnel: w272 -> [w274 _]
              frame False {
                n152 = disable-structure shown="Enabled" {
                  disable-tunnel: w274 -> [w275 w276]
                  frame Disabled {
                    n153 = call "Window-Exporting 8bit videos.vi"("Input cluster"=w275) -> ()  [unwired: 11 in]
                  }
                  frame Enabled {
                    n154 = call "Functional acq video generator.vi"("Input cluster"=w276) -> ()  [unwired: 11 in]
                  }
                }
              }
              frame True {
              }
            }
          }
        }
        n155 = call <vilib>:"Unset Busy.vi"("error in (no error)"=w267) -> ()  [unwired: 10 in, 1 out]
      }
    }
    n156 = local read "Stop (ind)"() -> (w264:bool)
  }
  n157 = while {
    shift-right: [w283] -> _
    shift-left: w24 -> [w282]
    tunnel: w35 -> [w281]
    shift-right: [w280] -> _
    shift-left: _ -> [w279]
    tunnel: [w278] -> w10
    tunnel: w11 -> [w277]
    tunnel: [w277] -> w12
    stop <- w284 stop-if-true
    # "EVENT HANDLING LOOP"
    n158 = event shown="[3] \"Scrollbar\", \"Channel to load\": Value Change" {
      selector: _ -> [_ _ _ _ _ _ _ _ _ _ _ _ _ _ _ _ _ _]
      dyn-events: _ -> [_ _ _ _ _ _ _ _ _ _ _ _ _ _ _ _ _ _]
      timeout: 250 -> [_ _ _ _ _ _ _ _ _ _ _ _ _ _ _ _ _ _]
      tunnel: [w286 w292 _ _ _ _ _ _ _ _ _ _ _ _ _ _ _ w420] -> w284
      tunnel: [w290 w295 w306 w310 w324 w330 w338 w351 w365 w370 w375 w383 w388 w393 w396 w398 w415 w422] -> w283
      tunnel: w282 -> [w290 w295 w306 w312 w324 w330 w338 w353 w365 w370 w375 w383 w388 w393 w396 w400 w415 w422]
      tunnel: w281 -> [_ w293 _ w311 _ w331 _ w352 _ w369 _ _ _ w390 _ w404 _ w421]
      tunnel: [w289 w291 w307 w309 w323 w333 w337 w342 w362 w367 w371 FALSE FALSE w389 w395 w401 w414 w419] -> w280
      tunnel: w279 -> [w289 w291 w307 w309 w323 w333 w337 w342 w362 w367 _ w382 _ w389 w395 w401 w414 w419]
      tunnel: [w287 _ _ _ _ _ _ _ _ _ _ _ _ _ _ _ _ w418] -> w278
      tunnel: w277 -> [w288 _ _ _ _ _ _ _ _ _ _ _ _ _ _ _ _ w417]
      event Timeout {
        n159 = event-data() -> ()  [unwired: 1 in, 1 out]
        n160 = call "Funct Viewer-Bring to front.vi"() -> ()  [unwired: 12 in]
        n161 = global read "General Globals.vi" "Stop application"() -> (w286:bool)
        n162 = property class="VI"(reference=w288) -> ("FP.State"=w287:T38)  [unwired: 1 in, 2 out]
      }
      event Menu Selection (User) {
        n163 = event-data() -> ("ItemTag"=w294:string)  [unwired: 1 in]
        n164 = case shown="\"Close\"" w294 {
          tunnel: w293 -> [_ w296 _ _ w301 _ _ _]
          tunnel: [_ _ _ _ w300 _ _ _] -> w292
          frame Default {
          }
          frame "Load dataset" {
            n165 = call "Time series viewer-Event handler-Load dataset.vi"("queue"=w296) -> ()  [unwired: 11 in]
          }
          frame "Playback speed..." {
            n166 = call "Window-Playback speed entry.vi"() -> ("Frame rate set (fps)"=w297:dbl)  [unwired: 10 in, 1 out]
            n167 = local write "Frame rate set (fps)"(w297) -> ()
          }
          frame "Original speed (x1)" {
            n168 = flat-sequence {
              frame #0 {
                n169 = global write "gl_Time series viewer globals.vi" "Use manual FPS?"(FALSE ("Use manual FPS?")) -> ()
              }
              frame #1 {
                n170 = call "AVI playback timing control.vi"() -> ("Frame rate set OR original (fps)"=w299:dbl)  [unwired: 8 in, 3 out]
                n171 = local write "Frame rate set (fps)"(w299) -> ()
              }
            }
          }
          frame "Close" {
            n172 = call "Time series viewer-Event handler-Exit.vi"("Queue in"=w301) -> ("Exit"=w300:bool)  [unwired: 10 in]
            n173 = case shown="True" w300 {
              frame False {
              }
              frame True {
                n174 = local write "Stop"(TRUE ("Stop")) -> ()
              }
            }
          }
          frame "Export snippet" {
            "Export snippet" <- TRUE
          }
          frame "Export 8-bit video" {
            "Export vid" <- TRUE
          }
          frame "Export TIFF series" {
            "Export images" <- TRUE
          }
        }
      }
      event "Scrollbar", "Speed Graph": Shortcut Menu Selection (User) {
        n175 = event-data() -> ("ItemTag"=w308:string)  [unwired: 1 in]
        n176 = call "Time series viewer-Shortcut menu handler.vi"("ItemTag"=w308) -> ()  [unwired: 11 in]
      }
      event "Scrollbar": Value Change {
        n177 = event-data() -> ()  [unwired: 1 in, 6 out]
        n178 = disable-structure shown="Enabled" {
          disable-tunnel: w312 -> [w315 _]
          disable-tunnel: w311 -> [w314 w316]
          disable-tunnel: [w313 _] -> w310
          frame Enabled {
            n179 = call "Event case-Scrollbar value change.vi"("Tick count in"=w315, "Queue in"=w314) -> ("Tick count"=w313:u32)  [unwired: 8 in, 1 out]
          }
          frame Disabled {
            n180 = Lossy Enqueue Element(queue=w316, element=Speed_Viewer_States_enum."Scroll bar event" ("States")) -> ()  [unwired: 1 in, 4 out]
          }
        }
      }
      event "Speed Graph": Shortcut Menu Activation? {
        n181 = event-data() -> ("MenuRef"=w320:refnum<k9>)  [unwired: 1 in]
        n182 = call "FGV_Speed graph behaviour-Main viewer.vi"("Function"=Get-Set-Clear_Control."Get") -> ("Speed graph behaviour"=w319:T39)  [unwired: 9 in, 1 out]
        n183 = case shown="\"Scrolling data\", Default" w319 {
          tunnel: [bool[] [FALSE, TRUE] bool[] [TRUE, FALSE]] -> w318
          frame "Scrolling data", Default {
          }
          frame "Scrolling cursor" {
          }
        }
        n184 = for {
          tunnel: string[] ["scrolling cursor", "scrolling data"] -> [w329] mode=indexing
          tunnel: w320 -> [w328]
          tunnel: w318 -> [w327] mode=indexing
          n185 = Set Menu Item Info(6:w327, 7:w329, 11:w328) -> ()  [unwired: 4 in, 2 out]
        }
        n186 = event-data() -> ()  [unwired: 2 in, 1 out]
      }
      event "Speed Graph": Cursor Move; "Speed Graph": Cursor Release {
        n187 = event-data() -> ("CursRef"=w332:refnum<vi>)  [unwired: 1 in]
        n188 = call "Event case-Speed graph cursor moved.vi"("queue in"=w331, "Cursor in"=w332) -> ()  [unwired: 9 in, 1 out]
      }
      event "Speed Graph": event type 3.0.x80000027 {
        n189 = event-data() -> ()  [unwired: 1 in, 1 out]
        n190 = call "FGV_Speed graph behaviour-Main viewer.vi"("Function"=Get-Set-Clear_Control."Get") -> ("Speed graph behaviour"=w335:T39)  [unwired: 9 in, 1 out]
        n191 = case shown="\"Scrolling data\", Default" w335 {
          tunnel: [TRUE FALSE] -> w334
          frame "Scrolling data", Default {
            # "Moving the speed data graph's cursor manually is \nprevented when the mode is \"Scrolling data\"."
          }
          frame "Scrolling cursor" {
            # "Moving the speed data graph's cursor manually is \nallowed when the mode is \"Scrolling cursor\"."
          }
        }
        n192 = event-data("Discard?"=w334) -> ()  [unwired: 1 in, 1 out]
      }
      event "Extraction Cursors": Value Change {
        # "Do not use the left cursor's change event"
        # "Sets the main slider to the value of the extraction cursor that was moved."
        n193 = event-data() -> ("OldVal"=w350:cluster{i32, i32}, "NewVal"=w343:cluster{i32, i32})  [unwired: 1 in]
        n194 = Not Equal?(x=w350, y=w343) -> (x != y?=w344:cluster{bool, bool})
        n195 = Unbundle(w344) -> (w341:bool)  [unwired: 1 out]
        n196 = Unbundle(w343) -> (w349:i32, w348:i32)
        n197 = Select(t=w348, s=w341, f=w349) -> (s? t:f=w345:i32)
        n198 = flat-sequence {
          tunnel: w352 -> [w356]
          tunnel: w353 -> [w357]
          tunnel: [w357] -> w347
          tunnel: [w356] -> w346
          tunnel: w345 -> [w355]
          tunnel: w341 -> [w354]
          tunnel: [w358] -> w351
          tunnel: w347 -> [w360]
          tunnel: w346 -> [w359]
          frame #0 {
            n199 = call "Sync scrollbars.vi"("Min cursor moved"=w354, "Scrollbar value"=w355) -> ()  [unwired: 9 in, 1 out]
          }
          frame #1 {
            n200 = call "Event case-Scrollbar value change.vi"("Tick count in"=w360, "Queue in"=w359) -> ("Tick count"=w358:u32)  [unwired: 8 in, 1 out]
          }
        }
      }
      event Value Change {
        n201 = event-data() -> ()  [unwired: 1 in, 6 out]
        n202 = call "Prepare image colour.vi"("Left Image Palette"="Colour") -> ("Color Palette"=w363:cluster{"Red":u8, "Green":u8, "Blue":u8}[], "Palette Type"=w364:u32)  [unwired: 8 in, 1 out]
        n203 = property on="Image" class="ImageControl"("Palette Type"=w364, "User Palette"=w363) -> ()  [unwired: 2 in, 2 out]
      }
      event "Experiment Path", "Number of rows to generate": Value Change {
        n204 = event-data() -> ()  [unwired: 1 in, 1 out]
        n205 = Enqueue Element At Opposite End(queue=w369, element=Speed_Viewer_States_enum."Initialise") -> ()  [unwired: 2 in, 3 out]
        n206 = local write "Stop"(TRUE ("Stop")) -> ()
      }
      event "Cams.Vid 1", "Cams.Vid 2", "Cams.Vid 3", "Cams.Vid 4": Mouse Down {
        # "http://zone.ni.com/reference/en-XX/help/371361K-01/lvhowto/drag_and_drop_programmatic_prepare/"
        # "Detects and registers when the mouse is clicked \nwithin the boundaries of a CamVid display. This allows to generate a \"Drag leave\" event for those displays (in a separate event case / Mouse leave case).\nThis is necessary because the Drag-Leave event does not work for this type of control."
        n207 = event-data() -> ("Button"=w372:u16, "Mods.Double Click"=w374:bool, "CtlRef"=w373:refnum<vi>)  [unwired: 1 in]
        n208 = case shown="True" w374 {
          tunnel: w372 -> [_ w377]
          tunnel: w373 -> [_ w379]
          frame False {
          }
          frame True {
            n209 = property class="ImageControl"(reference=w379) -> ("Label.Text"=w378:string)  [unwired: 1 in, 2 out]
            n210 = call "Open expanded image window.vi"("Button"=w377, "Image name"=w378) -> ()  [unwired: 10 in]
          }
        }
        n211 = case shown="1" w372 {
          tunnel: [_ TRUE] -> w371
          frame 0, Default {
          }
          frame 1 {
          }
        }
      }
      event "Cams.Vid 1", "Cams.Vid 2", "Cams.Vid 3", "Cams.Vid 4": Mouse Leave {
        n212 = event-data() -> ("CtlRef"=w380:refnum<vi>)  [unwired: 1 in]
        n213 = case shown="False" w382 {
          tunnel: w380 -> [_ w386]
          frame False {
          }
          frame True {
            n214 = property class="ImageControl"(reference=w386) -> ("Label.Text"=w384:string)  [unwired: 1 in, 2 out]
            n215 = call "Open expanded image window.vi"("Button"=u16 0, "Image name"=w384) -> ()  [unwired: 10 in]
          }
        }
      }
      event Mouse Up {
        n216 = event-data() -> ()  [unwired: 1 in, 1 out]
      }
      event "Back": Value Change {
        n217 = event-data() -> ()  [unwired: 1 in, 1 out]
        n218 = Enqueue Element At Opposite End(queue=w390, element=Speed_Viewer_States_enum."Back to start") -> ()  [unwired: 2 in, 3 out]
        n219 = local write "Stop"(TRUE ("Stop")) -> ()
      }
      event Value Change {
        n220 = event-data() -> ()  [unwired: 1 in, 1 out]
        n221 = global write "gl_Time series viewer globals.vi" "Intensity"("Intensity") -> ()
        n222 = call "16-bit display mapping.vi"() -> ()  [unwired: 11 in, 1 out]
      }
      event "Play": Value Change {
        n223 = event-data() -> ()  [unwired: 1 in, 1 out]
        n224 = flat-sequence {
          tunnel: w404 -> [w408]
          tunnel: [w408] -> w403
          tunnel: w400 -> [w405]
          tunnel: [w405] -> w399
          tunnel: w403 -> [w410]
          tunnel: [w410] -> w402
          tunnel: w399 -> [w409]
          tunnel: [w409] -> w397
          tunnel: w402 -> [w412]
          tunnel: [w411] -> w398
          tunnel: w397 -> [w411]
          frame #0 {
            n225 = local write "Stop"(FALSE ("Stop")) -> ()
            n226 = call "Set Play-Stop buttons.vi"("Function"=Select_Play-Stop_button_to_show."Show Stop button") -> ()  [unwired: 10 in, 1 out]
          }
          frame #1 {
            n227 = call "Set scrollbar at start.vi"("Queue in"=w410) -> ()  [unwired: 10 in, 1 out]
          }
          frame #2 {
            n228 = Enqueue Element(queue=w412, element=Speed_Viewer_States_enum."Playback" ("States")) -> ()  [unwired: 2 in, 3 out]
          }
        }
      }
      event "Stop": Value Change {
        n229 = event-data() -> ()  [unwired: 1 in, 1 out]
      }
      event Panel Close? {
        # "The panel close is always discarded here because it is closed conditionally in the yellow \"Save Windows Bounds\" vi."
        n230 = event-data() -> ()  [unwired: 1 in, 1 out]
        n231 = call "Time series viewer-Event handler-Exit.vi"("Queue in"=w421) -> ("Exit"=w420:bool)  [unwired: 10 in]
        n232 = case shown="True" w420 {
          frame False {
          }
          frame True {
            n233 = local write "Stop"(TRUE ("Stop")) -> ()
            n234 = global write "gl_Time series viewer globals.vi" "Close larger image windows"(TRUE ("Close larger image window")) -> ()
          }
        }
        n235 = property class="VI"(reference=w417) -> ("FP.State"=w418:T38)  [unwired: 1 in, 2 out]
        n236 = event-data("Discard?"=TRUE) -> ()  [unwired: 1 in, 1 out]
      }
    }
  }
  n237 = call "Funct Viewer-cleanup.vi"("error in (no error)"=w32, "I16 image ref"=w36) -> ("error out"=w9:errorcluster)  [unwired: 9 in]
  n238 = flat-sequence {
    tunnel: w14 -> [w428]
    tunnel: w12 -> [w426]
    tunnel: w10 -> [w427]
    tunnel: w9 -> [_]
    tunnel: w7 -> [_]
    frame #0 {
      n239 = disable-structure shown="Enabled" {
        disable-tunnel: [w429 FALSE ("Front Panel Window:Open")] -> w425
        frame Disabled {
          n240 = call <userlib>:"Detect_Application_Kind.vi"() -> ("Development System"=w430:bool)  [unwired: 9 in, 2 out]
          n241 = case shown="True" w430 {
            tunnel: [_ TRUE ("Front Panel Window:Open")] -> w429
            frame False {
            }
            frame True {
            }
          }
        }
        frame Enabled {
        }
      }
      n242 = call "Save_Windows_Bounds.vi"("FP.State"=w427, "Window Name (i.e. Key)"=w428, "Front Panel Window:Open"=w425, "Window VI's Ref"=w426) -> ()  [unwired: 7 in, 1 out]
    }
  }
